vi "GetLowPrioritySensors.vi"() -> ()   [LabVIEW 2019]
doc: "All low priority sensor reads should be placed in this VI."
uses:
  refnums.vi
  GRNF_AI.vi
  GRNF_Compressor.vi
  sensors.vi
  GRNF_CTREMotor.vi
  <vilib>/Rock Robotics/WPI/ThirdParty/Phoenix-LabVIEW/Motor Controller/Get/CTRE_Phoenix_MotorController_GetTemperature.vi
  robotprofile.vi
  <vilib>/Rock Robotics/WPI/ThirdParty/Phoenix-LabVIEW/Motor Controller/Get/CTRE_Phoenix_MotorController_GetVoltage.vi
panel:
  out "Pressure Change (psi/min)":dbl
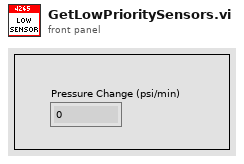
[diagram p1: front panel]
types:
  T1 = typedef "WPI_MotorControlDeviceRef.ctl" = cluster{"DeviceStatus":errorcluster, "Type":T2, "PWM":cluster{"PWM Channel":T3, "DeadBand":T4}, "CAN":cluster{"Device Number":u8, "SetOutput VI Ref":variant, "GetOutput VI Ref":variant, "Enable VI Ref":variant, "Disable VI Ref":variant, "Data":variant}, "Invert":bool, "DIO PWM":cluster{"PWM \"Enable\" Channel":T3, "DIOChannel":T5, "PWM Rate":dbl}}
  T2 = typedef "WPI_MotorControlType.ctl" = enum16{"PWM", "CAN", "DIO PWM"}
  T3 = typedef "FPGA_DIOPWMChannel.ctl" = enum8{"PWM 0", "PWM 1", "PWM 2", "PWM 3", "PWM 4", "PWM 5", "PWM 6", "PWM 7", "PWM 8", "PWM 9", "PWM MXP 0", "PWM MXP 1", "PWM MXP 2", "PWM MXP 3", "PWM MXP 4", "PWM MXP 5", "PWM MXP 6", "PWM MXP 7", "PWM MXP 8", "PWM MXP 9", "Invalid"}
  T4 = typedef "WPI_PWMDeadband.ctl" = cluster{"Name":string, "maxPositivePwm":i32, "minPositivePwm":i32, "centerPwm":i32, "maxNegativePwm":i32, "minNegativePwm":i32, "angularRange":u16}
  T5 = typedef "FPGA_DIOChannel.ctl" = enum8{"DIO 0", "DIO 1", "DIO 2", "DIO 3", "DIO 4", "DIO 5", "DIO 6", "DIO 7", "DIO 8", "DIO 9", "DIO MXP 0", "DIO MXP 1", "DIO MXP 2", "DIO MXP 3", "DIO MXP 4", "DIO MXP 5", "DIO MXP 6", "DIO MXP 7", "DIO MXP 8", "DIO MXP 9", "DIO MXP 10", "DIO MXP 11", "DIO MXP 12", "DIO MXP 13", "DIO MXP 14", "DIO MXP 15", "SPI Port CS1", "SPI Port CS2", "SPI Port CS3", "SPI Port MISO", "SPI Port MOSI", "Invalid"}
  T6 = typedef "WPI_CompressorDevRef.ctl" = cluster{"DevStatus":errorcluster, "Pneumatics Control Module":u8}
  T7 = typedef "WPI_AnalogChannelDevRef.ctl" = cluster{"DevStatus":errorcluster, "Analog Channel":T8}
  T8 = typedef "FPGA_AIChannel.ctl" = enum8{"AI 0", "AI 1", "AI 2", "AI 3", "AI MXP 0", "AI MXP 1", "AI MXP 2", "AI MXP 3", "Invalid"}
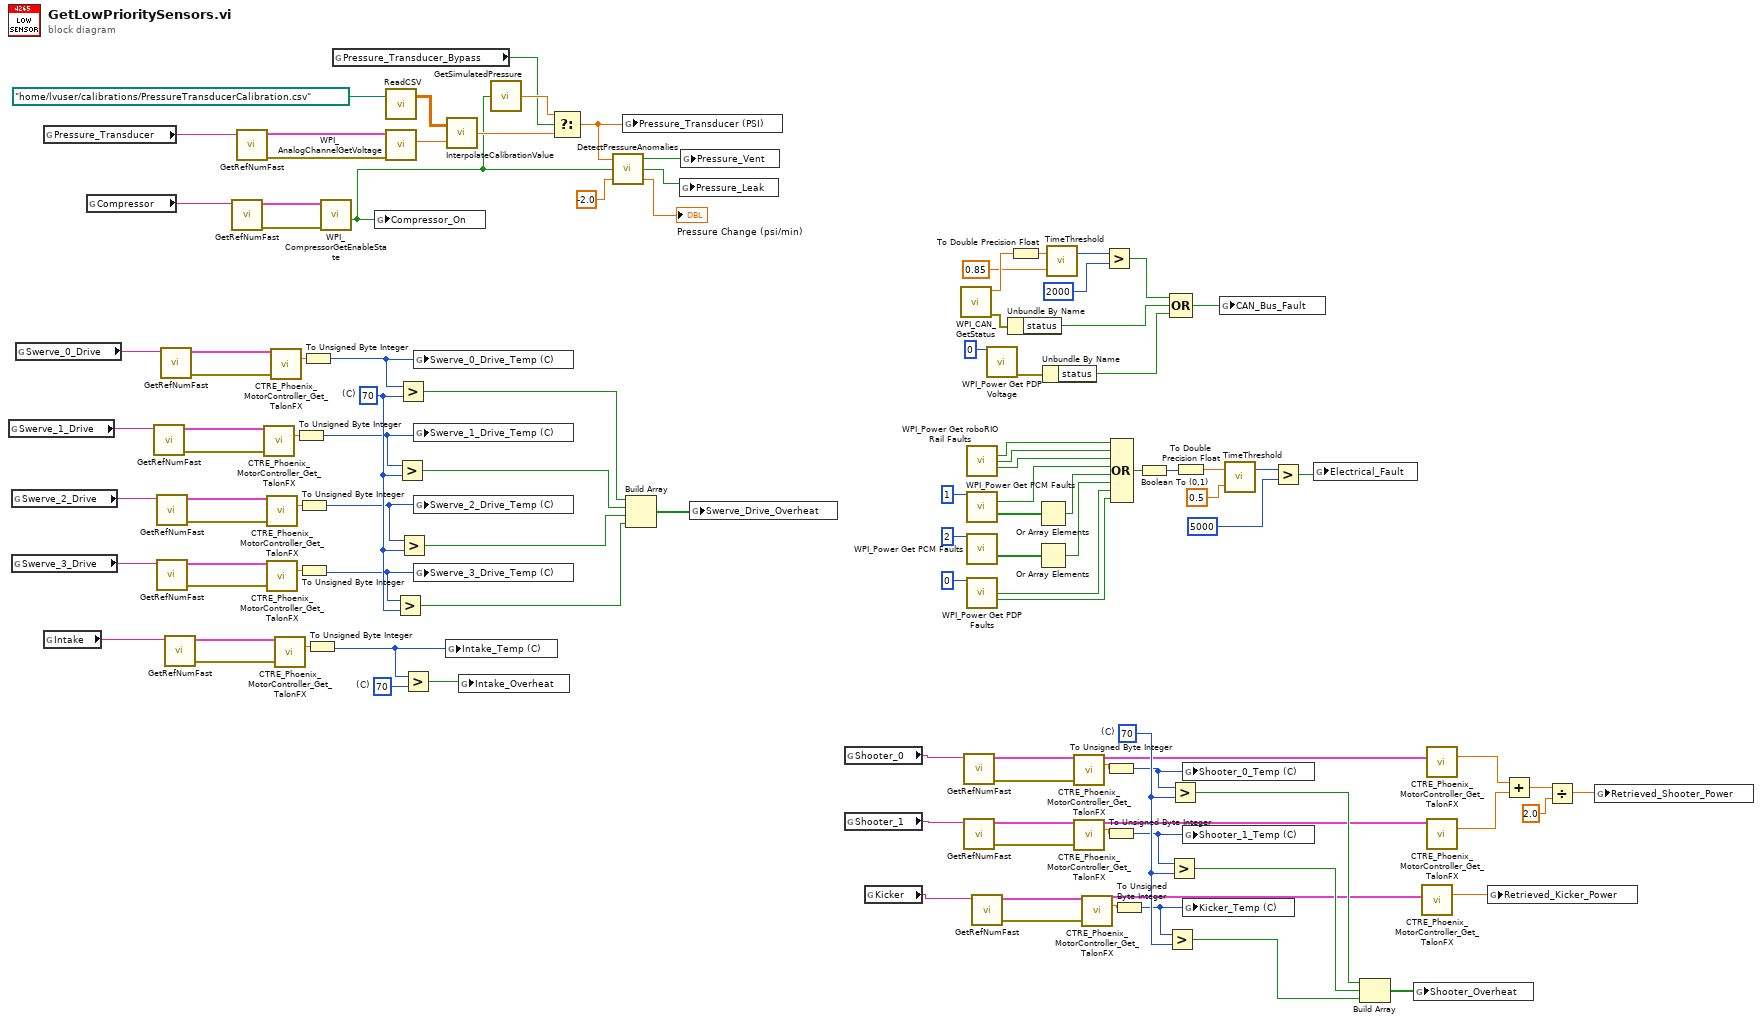
[diagram p0: block diagram]
diagram:
  w8 = u8 70  # (C)
  w40 = u8 70  # (C)
  w107 = u8 70  # (C)
  n1 = global read "refnums.vi" "Swerve_1_Drive"() -> (w81:string)
  n2 = global read "refnums.vi" "Swerve_2_Drive"() -> (w77:string)
  n3 = global read "refnums.vi" "Swerve_3_Drive"() -> (w73:string)
  n4 = global read "refnums.vi" "Swerve_0_Drive"() -> (w97:string)
  n5 = global read "refnums.vi" "Pressure_Transducer"() -> (w98:string)
  n6 = global read "refnums.vi" "Intake"() -> (w13:string)
  n7 = global read "refnums.vi" "Compressor"() -> (w109:string)
  n8 = call-poly "GetRefNumFast.vi"("RefNum Name"=w81) -> ("Error"=w79:errorcluster, "Device Reference"=w80:T1)  [unwired: 5 in]
  n9 = call-poly "GetRefNumFast.vi"("RefNum Name"=w77) -> ("Error"=w75:errorcluster, "Device Reference"=w76:T1)  [unwired: 5 in]
  n10 = call-poly "GetRefNumFast.vi"("RefNum Name"=w73) -> ("Error"=w71:errorcluster, "Device Reference"=w72:T1)  [unwired: 5 in]
  n11 = call-poly "GetRefNumFast.vi"("RefNum Name"=w97) -> ("Error"=w84:errorcluster, "Device Reference"=w85:T1)  [unwired: 5 in]
  n12 = call-poly "GetRefNumFast.vi"("RefNum Name"=w13) -> ("Error"=w11:errorcluster, "Device Reference"=w12:T1)  [unwired: 5 in]
  n13 = call-poly "GetRefNumFast.vi"("RefNum Name"=w109) -> ("Error"=w101:errorcluster, "Device Reference"=w108:T6)  [unwired: 5 in]
  n14 = call-poly "GetRefNumFast.vi"("RefNum Name"=w98) -> ("Error"=w99:errorcluster, "Device Reference"=w100:T7)  [unwired: 5 in]
  n15 = call-poly <vilib>:"CTRE_Phoenix_MotorController_Get_TalonFX.vi"("PhoenixMotorControlDevRef"=w80, "error in"=w79) -> ("Temperature (C)"=w78:dbl)  [unwired: 11 in, 2 out]
  n16 = call-poly <vilib>:"CTRE_Phoenix_MotorController_Get_TalonFX.vi"("PhoenixMotorControlDevRef"=w76, "error in"=w75) -> ("Temperature (C)"=w74:dbl)  [unwired: 11 in, 2 out]
  n17 = call-poly <vilib>:"CTRE_Phoenix_MotorController_Get_TalonFX.vi"("PhoenixMotorControlDevRef"=w72, "error in"=w71) -> ("Temperature (C)"=w70:dbl)  [unwired: 11 in, 2 out]
  n18 = call-poly <vilib>:"CTRE_Phoenix_MotorController_Get_TalonFX.vi"("PhoenixMotorControlDevRef"=w85, "error in"=w84) -> ("Temperature (C)"=w83:dbl)  [unwired: 11 in, 2 out]
  n19 = call-poly <vilib>:"CTRE_Phoenix_MotorController_Get_TalonFX.vi"("PhoenixMotorControlDevRef"=w12, "error in"=w11) -> ("Temperature (C)"=w10:dbl)  [unwired: 11 in, 2 out]
  n20 = To Unsigned Byte Integer(number=w78) -> (unsigned 8bit integer=w67:u8)
  n21 = To Unsigned Byte Integer(number=w74) -> (unsigned 8bit integer=w69:u8)
  n22 = To Unsigned Byte Integer(number=w70) -> (unsigned 8bit integer=w68:u8)
  n23 = To Unsigned Byte Integer(number=w83) -> (unsigned 8bit integer=w82:u8)
  n24 = To Unsigned Byte Integer(number=w10) -> (unsigned 8bit integer=w9:u8)
  n25 = call <vilib>:"WPI_CompressorGetEnableState.vi"("error in (no error)"=w101, "CompressorDevRef"=w108) -> ("Compressor Running"=w3:bool)  [unwired: 6 in, 3 out]
  n26 = global read "robotprofile.vi" "Pressure_Transducer_Bypass"() -> (w43:bool)
  n27 = global write "sensors.vi" "Compressor_On"(w3) -> ()
  n28 = call "ReadCSV.vi"("File Path (.csv)"=path "/home/lvuser/calibrations/PressureTransducerCalibration.csv" ("path")) -> ("Data (index by row)"=w111:dbl[][])  [unwired: 1 in, 1 out]
  n29 = call <vilib>:"WPI_AnalogChannelGetVoltage.vi"("error in (no error)"=w99, "AIDeviceRef"=w100) -> ("Voltage"=w110:dbl)  [unwired: 7 in, 2 out]
  n30 = Greater?(x=w68, y=w107) -> (0:w103:bool)
  n31 = Greater?(x=w67, y=w107) -> (0:w105:bool)
  n32 = Greater?(x=w82, y=w107) -> (0:w106:bool)
  n33 = Greater?(x=w69, y=w107) -> (0:w104:bool)
  n34 = Greater?(x=w9, y=w8) -> (0:w7:bool)
  n35 = global write "sensors.vi" "Swerve_0_Drive_Temp (C)"(w82) -> ()
  n36 = global write "sensors.vi" "Swerve_1_Drive_Temp (C)"(w67) -> ()
  n37 = global write "sensors.vi" "Swerve_2_Drive_Temp (C)"(w69) -> ()
  n38 = global write "sensors.vi" "Swerve_3_Drive_Temp (C)"(w68) -> ()
  n39 = global write "sensors.vi" "Intake_Temp (C)"(w9) -> ()
  n40 = call "InterpolateCalibrationValue.vi"("Input"=w110, "Calibration Data"=w111) -> ("Interpolated Output"=w44:dbl)
  n41 = global write "sensors.vi" "Intake_Overheat"(w7) -> ()
  n42 = call "GetSimulatedPressure.vi"("Compressor On"=w3) -> ("Simulated Pressure Transducer"=w45:dbl)
  n43 = Select(t=w45, s=w43, f=w44) -> (s? t:f=w2:dbl)
  n44 = call "DetectPressureAnomalies.vi"("Pressure Loss Threshold (psi/min)"=-2.0, "Compressor Running"=w3, "Pressure (psi)"=w2) -> ("Pressure Change (psi/min)"=→"Pressure Change (psi/min)":dbl, "Pressure Leak"=w6:bool, "Pressure Vent"=w5:bool)
  n45 = global write "sensors.vi" "Pressure_Transducer (PSI)"(w2) -> ()
  n46 = Build Array(w106, w105, w104, w103) -> (w102:bool[])
  n47 = global write "sensors.vi" "Pressure_Leak"(w6) -> ()
  n48 = global write "sensors.vi" "Pressure_Vent"(w5) -> ()
  n49 = global write "sensors.vi" "Swerve_Drive_Overheat"(w102) -> ()
  n50 = global read "refnums.vi" "Shooter_0"() -> (w28:string)
  n51 = global read "refnums.vi" "Shooter_1"() -> (w27:string)
  n52 = global read "refnums.vi" "Kicker"() -> (w26:string)
  n53 = call <vilib>:"WPI_CAN_GetStatus.vi"() -> ("error out"=w66:errorcluster, "Percent Bus Utilization"=w58:sgl)  [unwired: 6 in, 4 out]
  n54 = call-poly "GetRefNumFast.vi"("RefNum Name"=w28) -> ("Error"=w36:errorcluster, "Device Reference"=w37:T1)  [unwired: 5 in]
  n55 = call-poly "GetRefNumFast.vi"("RefNum Name"=w27) -> ("Error"=w33:errorcluster, "Device Reference"=w34:T1)  [unwired: 5 in]
  n56 = call <vilib>:"WPI_Power Get roboRIO Rail Faults.vi"() -> ("3.3V User Rail Short"=w96:bool, "5 V User Rail Short"=w95:bool, "6 V User Rail Short"=w94:bool)  [unwired: 10 in, 3 out]
  n57 = call <vilib>:"WPI_Power Get PCM Faults.vi"("Pneumatics Control Module (0)"=u8 1) -> ("Compressor Fault"=w93:bool, "All Solenoid Faults"=w91:bool[])  [unwired: 11 in, 2 out]
  n58 = call <vilib>:"WPI_Power Get PCM Faults.vi"("Pneumatics Control Module (0)"=u8 2) -> ("All Solenoid Faults"=w89:bool[])  [unwired: 11 in, 3 out]
  n59 = call <vilib>:"WPI_Power Get PDP Faults.vi"("Power Distribution Panel (0)"=u8 0) -> ("Temperature Fault"=w62:bool, "Hardware Fault"=w61:bool)  [unwired: 10 in, 3 out]
  n60 = call-poly "GetRefNumFast.vi"("RefNum Name"=w26) -> ("Error"=w30:errorcluster, "Device Reference"=w31:T1)  [unwired: 5 in]
  n61 = call <vilib>:"WPI_Power Get PDP Voltage.vi"("Power Distribution Panel (0)"=u8 0) -> ("error out"=w60:errorcluster)  [unwired: 13 in, 1 out]
  n62 = Unbundle By Name(w66) -> ("status"=w65:bool)
  n63 = To Double Precision Float(number=w58) -> (double precision float=w56:dbl)
  n64 = Or Array Elements(Boolean array=w91) -> (logical OR=w90:bool)
  n65 = Or Array Elements(Boolean array=w89) -> (logical OR=w87:bool)
  n66 = Unbundle By Name(w60) -> ("status"=w59:bool)
  n67 = call "TimeThreshold.vi"("Threshold"=0.85, "Current Value"=w56) -> ("Time Above Threshold (ms)"=w55:u32)  [unwired: 1 out]
  n68 = call-poly <vilib>:"CTRE_Phoenix_MotorController_Get_TalonFX.vi"("PhoenixMotorControlDevRef"=w37, "error in"=w36) -> ("PhoenixMotorControlDevRef"=w17:T1, "Temperature (C)"=w35:dbl)  [unwired: 11 in, 1 out]
  n69 = call-poly <vilib>:"CTRE_Phoenix_MotorController_Get_TalonFX.vi"("PhoenixMotorControlDevRef"=w34, "error in"=w33) -> ("PhoenixMotorControlDevRef"=w16:T1, "Temperature (C)"=w32:dbl)  [unwired: 11 in, 1 out]
  n70 = call-poly <vilib>:"CTRE_Phoenix_MotorController_Get_TalonFX.vi"("PhoenixMotorControlDevRef"=w31, "error in"=w30) -> ("PhoenixMotorControlDevRef"=w14:T1, "Temperature (C)"=w29:dbl)  [unwired: 11 in, 1 out]
  n71 = Greater?(x=w55, y=u32 2000) -> (0:w53:bool)
  n72 = To Unsigned Byte Integer(number=w35) -> (unsigned 8bit integer=w25:u8)
  n73 = To Unsigned Byte Integer(number=w32) -> (unsigned 8bit integer=w24:u8)
  n74 = Compound Arithmetic op=OR(w96, w95, w94, w93, w90, w87, w62, w61) -> (w52:bool)
  n75 = To Unsigned Byte Integer(number=w29) -> (unsigned 8bit integer=w23:u8)
  n76 = Boolean To (0,1)(Boolean=w52) -> (0, 1=w51:i16)
  n77 = Greater?(x=w23, y=w40) -> (0:w39:bool)
  n78 = Greater?(x=w24, y=w40) -> (0:w41:bool)
  n79 = Compound Arithmetic op=OR(w53, w65, w59) -> (w63:bool)
  n80 = Greater?(x=w25, y=w40) -> (0:w42:bool)
  n81 = To Double Precision Float(number=w51) -> (double precision float=w50:dbl)
  n82 = global write "sensors.vi" "Shooter_0_Temp (C)"(w25) -> ()
  n83 = global write "sensors.vi" "Shooter_1_Temp (C)"(w24) -> ()
  n84 = global write "sensors.vi" "Kicker_Temp (C)"(w23) -> ()
  n85 = global write "sensors.vi" "CAN_Bus_Fault"(w63) -> ()
  n86 = call "TimeThreshold.vi"("Threshold"=0.5, "Current Value"=w50) -> ("Time Above Threshold (ms)"=w48:u32)  [unwired: 1 out]
  n87 = Greater?(x=w48, y=u32 5000) -> (0:w46:bool)
  n88 = global write "sensors.vi" "Electrical_Fault"(w46) -> ()
  n89 = Build Array(w42, w41, w39) -> (w38:bool[])
  n90 = global write "sensors.vi" "Shooter_Overheat"(w38) -> ()
  n91 = call-poly <vilib>:"CTRE_Phoenix_MotorController_Get_TalonFX.vi"("PhoenixMotorControlDevRef"=w14) -> ("Percent Output"=w15:dbl)  [unwired: 10 in, 4 out]
  n92 = call-poly <vilib>:"CTRE_Phoenix_MotorController_Get_TalonFX.vi"("PhoenixMotorControlDevRef"=w17) -> ("Percent Output"=w19:dbl)  [unwired: 10 in, 4 out]
  n93 = call-poly <vilib>:"CTRE_Phoenix_MotorController_Get_TalonFX.vi"("PhoenixMotorControlDevRef"=w16) -> ("Percent Output"=w18:dbl)  [unwired: 10 in, 4 out]
  n94 = global write "sensors.vi" "Retrieved_Kicker_Power"(w15) -> ()
  n95 = Add(x=w19, y=w18) -> (x+y=w21:dbl)
  n96 = Divide(x=w21, y=2.0) -> (x/y=w20:dbl)
  n97 = global write "sensors.vi" "Retrieved_Shooter_Power"(w20) -> ()
